vi "TempHumiditySensorV2_1.vi"() -> ()   [LabVIEW 2024]
uses:
  Driver/Public/Digital Pull Direction.ctl
  4d20a38f-85d9-49a3-8b57-4ea18b2081fb.vi
  f2578fff-0ee8-48cd-a801-9939c6f2dcf5.vi
  Driver/CTIPicoVISA.lvlib
panel:
  out "Humidity":dbl(slide) scale=0.0..100.0
  out "Thermometer":dbl(slide) scale=0.0..100.0
  out "Data":string
  out "TimedOut":bool
  out "Humidity":dbl(graph)
  out "Temperature":dbl(graph)
  in  "Grove Connector":enum16{"I2C0", "I2C1"}(ring)
  in  "VISA resource name in":refnum<visa-resource-name>="COM10"
  out "LoopIndex":i32
  in  "Stop":bool
  out "Identity":T1
  # "https://wiki.seeedstudio.com/Grove-Temperature-Humidity-Sensor-DH20/"
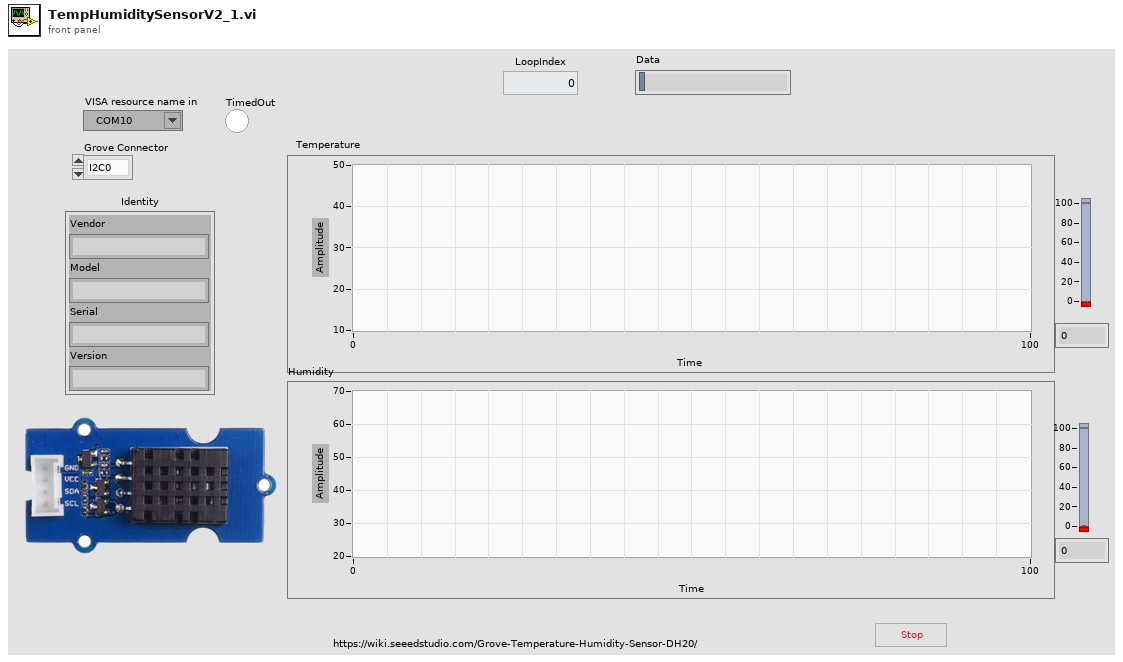
[diagram p1: front panel]
types:
  T1 = cluster{"Vendor":string, "Model":string, "Serial":string, "Version":string}
  T2 = typedef "CTIPicoVISA.lvlib/Digital Pull Direction.ctl" = enum16{"None", "Up", "Down", "Both"}
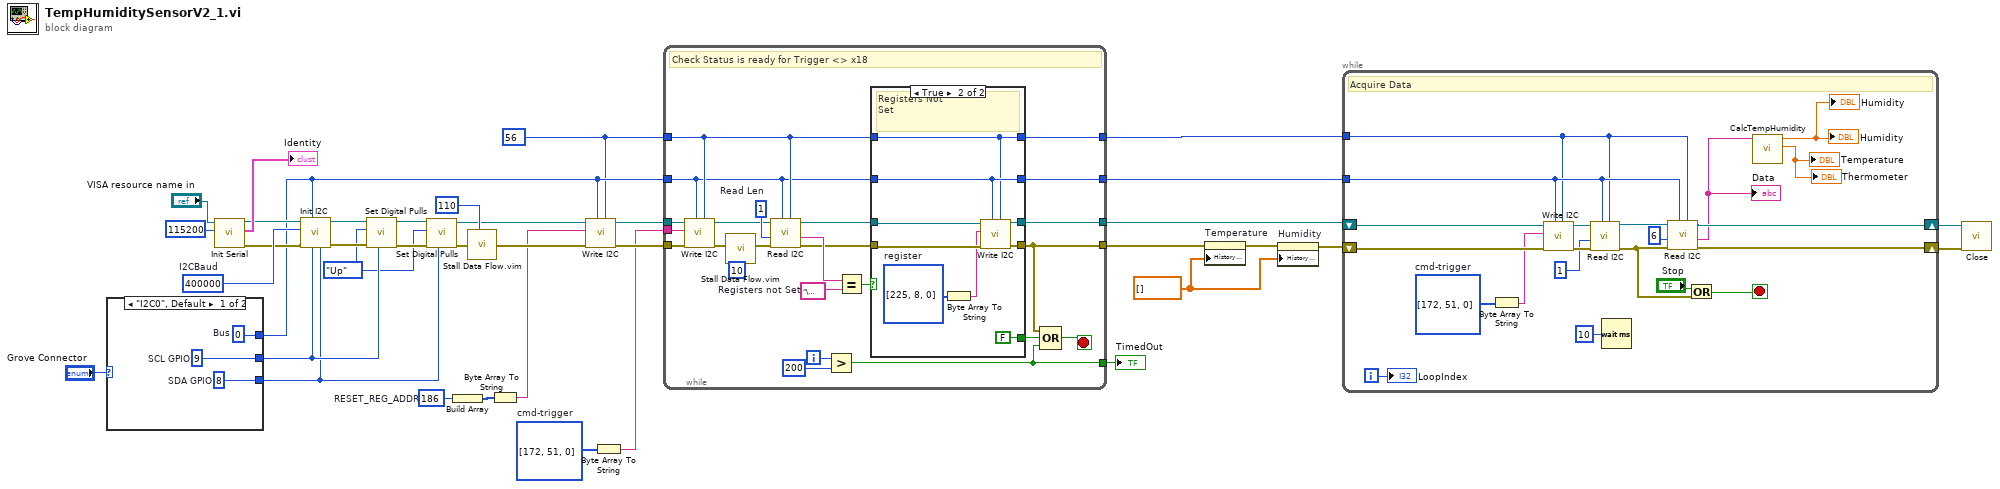
[diagram p0: block diagram]
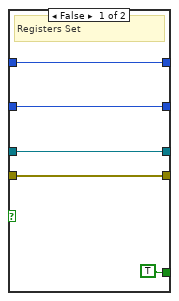
[diagram p2: hidden frame]
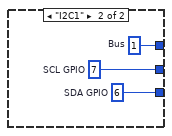
[diagram p3: hidden frame]
diagram:
  w2 = u8[] [172, 51, 0]  # cmd-trigger
  w16 = dbl[] [] ("History Data")
  w26 = Digital_Pull_Direction."Up" ("Pull")
  w33 = u32 400000  # I2CBaud
  w37 = u8 186  # RESET_REG_ADDR
  w4 = u8 56 ("Address")
  n1 = case shown="\"I2C0\", Default" "Grove Connector" {
    tunnel: [w40 w43] -> w27
    tunnel: [w39 w42] -> w25
    tunnel: [w38 w41] -> w5
    frame "I2C0", Default {
      w38 = u8 0  # Bus
      w39 = 8  # SDA GPIO
      w40 = 9  # SCL GPIO
    }
    frame "I2C1" {
      w41 = u8 1  # Bus
      w42 = 6  # SDA GPIO
      w43 = 7  # SCL GPIO
    }
  }
  n2 = call "Init Serial.vi"("Baud (115200)"=u32 115200, "VISA resource name in"="VISA resource name in") -> ("error out"=w21:errorcluster, "Identity"=→"Identity":T1, "VISA resource name Out"=w22:refnum<visa-resource-name>)  [unwired: 7 in]
  n3 = call "Init I2C.vi"("SDA GPIO"=w25, "SCL GPIO"=w27, "Bus"=w5, "error in (no error)"=w21, "Baud"=w33, "VISA resource name in"=w22) -> ("error out"=w30:errorcluster, "VISA resource name"=w31:refnum<visa-resource-name>)  [unwired: 4 in]
  n4 = call "Set Digital Pulls.vi"("GPIO"=w27, "error in (no error)"=w30, "Pull"=w26, "VISA resource name in"=w31) -> ("error out"=w28:errorcluster, "VISA resource name"=w29:refnum<visa-resource-name>)  [unwired: 6 in]
  n5 = call "Set Digital Pulls.vi"("GPIO"=w25, "error in (no error)"=w28, "Pull"=w26, "VISA resource name in"=w29) -> ("error out"=w23:errorcluster, "VISA resource name"=w7:refnum<visa-resource-name>)  [unwired: 6 in]
  n6 = Build Array(w37) -> (w36:u8[])
  n7 = call "Stall Data Flow.vim"("value in"=w23, "milliseconds to wait"=u32 110) -> ("value out"=w6:errorcluster)  [unwired: 1 out]
  n8 = Byte Array To String(unsigned byte array=w36) -> (string=w3:string)
  n9 = call "Write I2C.vi"("Address"=w4, "Bus"=w5, "error in (no error)"=w6, "Data"=w3, "VISA resource name in"=w7) -> ("error out"=w8:errorcluster, "VISA resource name"=w9:refnum<visa-resource-name>)  [unwired: 5 in]
  n10 = Byte Array To String(unsigned byte array=w2) -> (string=w1:string)
  n11 = while {
    tunnel: w4 -> [w48]
    tunnel: [w47] -> w14
    tunnel: w5 -> [w45]
    tunnel: [w44] -> w13
    tunnel: w8 -> [w67]
    tunnel: w9 -> [w66]
    tunnel: w1 -> [w65]
    tunnel: [w49] -> w10
    tunnel: [w51] -> w11
    tunnel: [w54] -> w12
    i -> [w57]
    stop <- w55 stop-if-true
    w58 = "\u0018"  # Registers not Set
    w62 = u8 1  # Read Len
    # "Check Status is ready for Trigger <> x18"
    n12 = call "Write I2C.vi"("Address"=w48, "Bus"=w45, "error in (no error)"=w67, "Data"=w65, "VISA resource name in"=w66) -> ("error out"=w64:errorcluster, "VISA resource name"=w60:refnum<visa-resource-name>)  [unwired: 5 in]
    n13 = call "Stall Data Flow.vim"("value in"=w64, "milliseconds to wait"=u32 10) -> ("value out"=w61:errorcluster)  [unwired: 1 out]
    n14 = call "Read I2C.vi"("Address"=w48, "Bus"=w45, "error in (no error)"=w61, "Len"=w62, "VISA resource name in"=w60) -> ("error out"=w50:errorcluster, "Data"=w59:string, "VISA resource name"=w52:refnum<visa-resource-name>)  [unwired: 4 in]
    n15 = Greater?(x=w57, y=200) -> (0:w54:bool)
    n16 = Equal?(x=w59, y=w58) -> (x = y?=w53:bool)
    n17 = case shown="True" w53 {
      tunnel: w52 -> [w70 w78]
      tunnel: [w70 w79] -> w51
      tunnel: w50 -> [w69 w77]
      tunnel: [w69 w80] -> w49
      tunnel: w48 -> [w72 w75]
      tunnel: [w72 w75] -> w47
      tunnel: [TRUE FALSE] -> w46
      tunnel: w45 -> [w71 w76]
      tunnel: [w71 w76] -> w44
      frame False {
        # "Registers Set"
      }
      frame True {
        w74 = u8[] [225, 8, 0]  # register
        # "Registers Not\nSet"
        n18 = Byte Array To String(unsigned byte array=w74) -> (string=w73:string)
        n19 = call "Write I2C.vi"("Address"=w75, "Bus"=w76, "error in (no error)"=w77, "Data"=w73, "VISA resource name in"=w78) -> ("error out"=w80:errorcluster, "VISA resource name"=w79:refnum<visa-resource-name>)  [unwired: 5 in]
      }
    }
    n20 = Compound Arithmetic op=OR(w49, w46, w54) -> (w55:bool)
  }
  "TimedOut" <- w12
  n21 = property on="Temperature" class="WFChart (strict)"(error in=w10, "History Data"=w16) -> (error out=w17:errorcluster)  [unwired: 1 in, 1 out]
  n22 = property on="Humidity" class="WFChart (strict)"(error in=w17, "History Data"=w16) -> (error out=w18:errorcluster)  [unwired: 1 in, 1 out]
  n23 = while {
    tunnel: w13 -> [w90]
    tunnel: w14 -> [w88]
    shift-right: [w87] -> w19
    shift-left: w18 -> [w102]
    shift-right: [w86] -> w20
    shift-left: w11 -> [w101]
    i -> [w99]
    stop <- w98 stop-if-true
    w93 = u8[] [172, 51, 0]  # cmd-trigger
    # "Acquire Data"
    n24 = Byte Array To String(unsigned byte array=w93) -> (string=w97:string)
    n25 = call "Write I2C.vi"("Address"=w88, "Bus"=w90, "error in (no error)"=w102, "Data"=w97, "VISA resource name in"=w101) -> ("error out"=w96:errorcluster, "VISA resource name"=w95:refnum<visa-resource-name>)  [unwired: 5 in]
    n26 = call "Read I2C.vi"("Address"=w88, "Bus"=w90, "error in (no error)"=w96, "Len"=u8 1 ("Read Len"), "VISA resource name in"=w95) -> ("error out"=w92:errorcluster, "VISA resource name"=w91:refnum<visa-resource-name>)  [unwired: 4 in, 1 out]
    n27 = Wait (ms)(milliseconds to wait=u32 10) -> ()  [unwired: 1 out]
    n28 = call "Read I2C.vi"("Address"=w88, "Bus"=w90, "error in (no error)"=w92, "Len"=u8 6 ("Read Len"), "VISA resource name in"=w91) -> ("error out"=w87:errorcluster, "Data"=w85:string, "VISA resource name"=w86:refnum<visa-resource-name>)  [unwired: 4 in]
    "Data" <- w85
    n29 = Or(x="Stop", y=w92) -> (x .or. y?=w98:bool)
    n30 = call "CalcTempHumidity.vi"("Data"=w85) -> ("Temperature (°C)"=→"Temperature" →"Thermometer":dbl, "RHumidity%"=→"Humidity" →"Humidity":dbl)  [unwired: 9 in]
    "LoopIndex" <- w99
  }
  n31 = call "Close.vi"("error in (no error)"=w19, "VISA resource name in"=w20) -> ()  [unwired: 9 in, 1 out]
